vi "Query Catalog.vi"(8 "error in (no error)":errorcluster {"code" format="%.0x"}, 9 "WaveformListBufferSize":i32=256, 11 "instrument handle":refnum<k15>) -> (0 "error out":errorcluster {"code" format="%.0x"}, 1 "MemoryFree":dbl, 2 "MemoryUsed":dbl, 3 "instrument handle out":refnum<k15>, 4 "NumberOfFiles":i32, 5 "WaveformList":string)   [LabVIEW 2009, in "Keysight XSAn.lvlib"]
doc: "Queries the test set for the list of waveform segments in the ARB memory.\n\nSupported Models: M8920A, M9420A, M9421A."
uses:
  <instrlib>/Keysight XSAn/Keysight XSAn.lvlib
  AgXSAn.dll
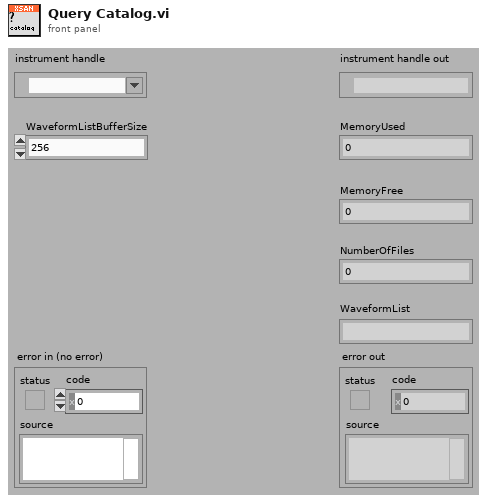
[diagram p1: front panel]
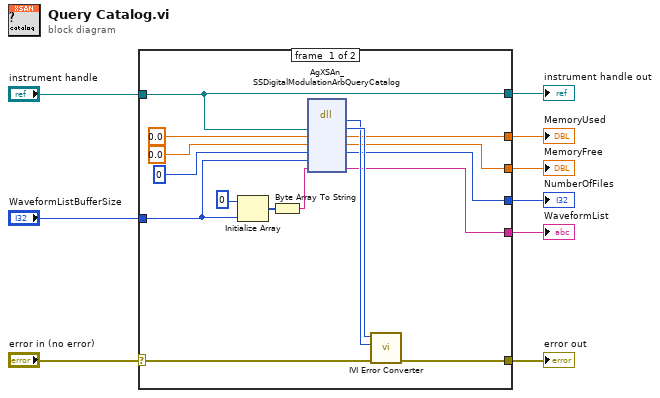
[diagram p0: block diagram]
diagram:
  n1 = case shown="No Error" "error in (no error)" {
    selector: "error in (no error)" -> [w23 w27]
    tunnel: [w22 w27] -> w9
    tunnel: "instrument handle" -> [w11 w26]
    tunnel: [w20 _] -> w6
    tunnel: [w18 _] -> w5
    tunnel: [w16 _] -> w4
    tunnel: "WaveformListBufferSize" -> [w10 _]
    tunnel: [w12 _] -> w2
    tunnel: [w11 w26] -> w1
    frame #0 {
      n2 = Initialize Array(u8 0 ("element"), w10) -> (w14:u8[])
      n3 = Byte Array To String(unsigned byte array=w14) -> (string=w15:string)
      n4 = dll-call lib="AgXSAn**.dll" fn="AgXSAn_SSDigitalModulationArbQueryCatalog"("Vi"=w11, "MemoryUsed"=0.0, "MemoryFree"=0.0, "NumberOfFiles"=0, "WaveformListBufferSize"=w10, "WaveformList"=w15) -> (w24:i32, "Vi"=w25:u32, "MemoryUsed"=w20:dbl, "MemoryFree"=w18:dbl, "NumberOfFiles"=w16:i32, "WaveformList"=w12:string)  [unwired: 4 in, 2 out]
      n5 = call <instrlib>:"IVI Error Converter.vi"("error in (no error)"=w23, "IVI error code (0)"=w24, "instrument handle"=w25) -> ("error out"=w22:errorcluster)  [unwired: 7 in, 1 out]
    }
    frame #1 {
    }
  }
  "error out" <- w9
  "instrument handle out" <- w1
  "MemoryUsed" <- w6
  "MemoryFree" <- w5
  "NumberOfFiles" <- w4
  "WaveformList" <- w2
